vi "CalInjRT.vi"(8 "error in (no error)":errorcluster, 11 "Boolean in":refnum<vi>) -> (0 "error out":errorcluster)   [LabVIEW 2016]
uses:
  controls/MotorStates.ctl
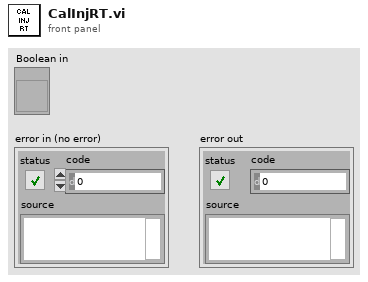
[diagram p1: front panel]
types:
  T1 = typedef "RT-Variables.lvlib/MotorStates.ctl" = enum16{"Open", "Close", "Moving"}
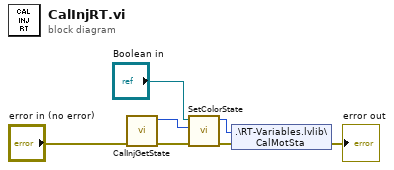
[diagram p0: block diagram]
diagram:
  n1 = call "CalInjGetState.vi"("error in (no error)"="error in (no error)") -> ("error out"=w2:errorcluster, "CalMotSta"=w1:T1)  [unwired: 9 in]
  n2 = call "SetColorState.vi"("error in (no error)"=w2, "MotorState"=w1, "Boolean in"="Boolean in") -> ("error out"=w5:errorcluster, "MotorState Out"=w4:T1)  [unwired: 6 in, 1 out]
  n3 = shared-variable ".\\RT-Variables.lvlib\\CalMotSta"(w4, error in=w5) -> (error out=→"error out":errorcluster)
